vi "Configure Pulse.vi"(4 "Delay (0.00 s)":dbl min=-1000000.0 max=1000000.0, 6 "Fall (20 ns)":dbl=2e-08 format="%#.3g", 7 "Duty (20%)":dbl=20.0 min=0.0001 max=100.0 format="%.4g", 8 "error in (no error)":errorcluster, 9 "Rise (20 ns)":dbl=2e-08 format="%#.3g", 10 "Channel (1:Channel 1)":i32(ring)=1 items=["Channel 1"=1, "Channel 2"=2], 11 "VISA resource name":refnum<visa-resource-name>) -> (0 "error out":errorcluster, 3 "VISA resource name out":refnum<visa-resource-name>)   [LabVIEW 2015, in "SDG X Series.lvlib"]
doc: "Configures the pulse waveform and parameters."
uses:
  <instrlib>/SDG X Series/SDG X Series.lvlib
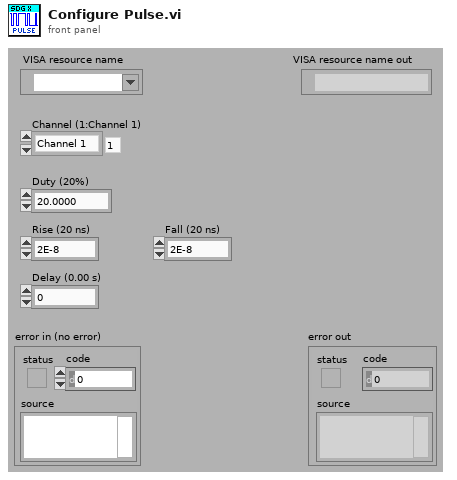
[diagram p1: front panel]
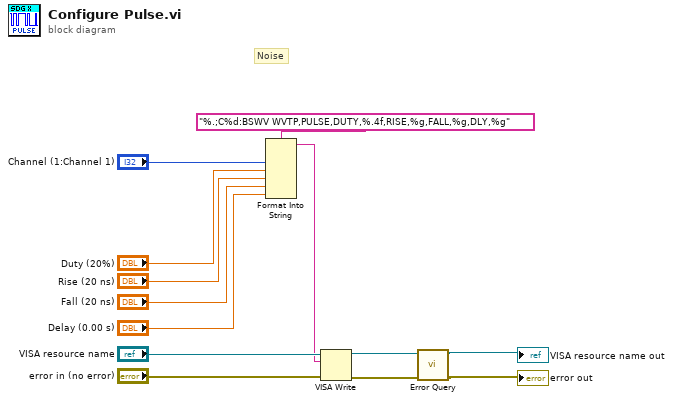
[diagram p0: block diagram]
diagram:
  # "Noise"
  n1 = Format Into String(format string="%.;C%d:BSWV WVTP,PULSE,DUTY,%.4f,RISE,%g,FALL,%g,DLY,%g", "Channel (1:Channel 1)", "Duty (20%)", "Rise (20 ns)", "Fall (20 ns)", "Delay (0.00 s)") -> (resulting string=w10:string)  [unwired: 2 in, 1 out]
  n2 = VISA Write(VISA resource name="VISA resource name", write buffer=w10, error in (no error)="error in (no error)") -> (VISA resource name out=w5:refnum<visa-resource-name>, error out=w4:errorcluster)  [unwired: 1 out]
  n3 = call <instrlib>:"Error Query.vi"("error in (no error)"=w4, "VISA resource name"=w5) -> ("error out"=→"error out":errorcluster, "VISA resource name out"=→"VISA resource name out":refnum<visa-resource-name>)  [unwired: 6 in, 2 out]
